vi "UI_Export Setting.vi"(8 "error in (no error)":errorcluster) -> (0 "error out":errorcluster)   [LabVIEW 2015, in "ConfigHelper.lvlib"]
uses:
  ConfigHelper.lvlib
  Control_Export File Setup.ctl
  Control_UI_Export Setting.ctl
  Control_UI_Export Setting State.ctl
  <vilib>/addons/PointValueMap/controls/PointMap.ctl
  <vilib>/addons/PointValueMap/PointValueMap.lvlib
panel:
  in  "Export File Setup":T1
  in  "Copy Device":bool
  in  "Save Button":bool
  in  "Import from TDMS":bool
  in  "Remove Channel":bool
  in  "Add Channel":bool
  in  "Remove Device":bool
  in  "Add Device":bool
  in  "Channel Names":i32[](listbox)
  in  "Device Name":i32[](listbox)
  in  "OK Button":bool
  in  "Cancel Button":bool
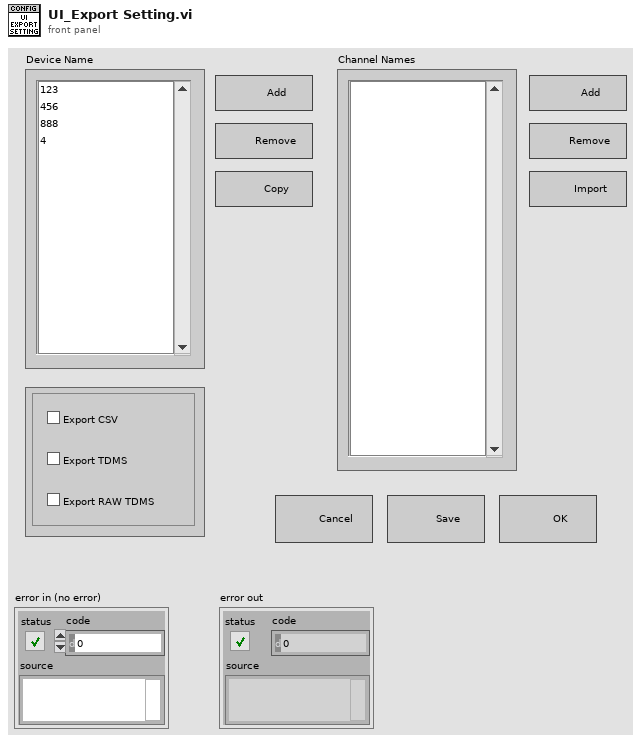
[diagram p1: front panel]
types:
  T1 = typedef "ConfigHelper.lvlib/Control_Export File Setup.ctl" = cluster{"CSV":bool, "TDMS":bool, "RAW TDMS":bool}
  T2 = typedef "ConfigHelper.lvlib/Control_UI_Export Setting State.ctl" = enum16{"Init", "Wait", "Exit", "Write to File", "Read from PVM", "Write to PVM", "Update Device", "Add Device", "Remove Device", "Copy Device", "Update Channel", "Add Channel", "Remove Channel", "Import from TDMS"}
  T3 = typedef "ConfigHelper.lvlib/Control_UI_Export Setting.ctl" = cluster{"State":T2, "Map":T4, "Device Name":refnum<vi>, "Channel Name":refnum<vi>, "File Setup":refnum<vi>, "Name":string, "Devices Selected":i32[]}
  T4 = typedef "PointValueMap.lvlib/PointMap.ctl" = refnum<data-value>
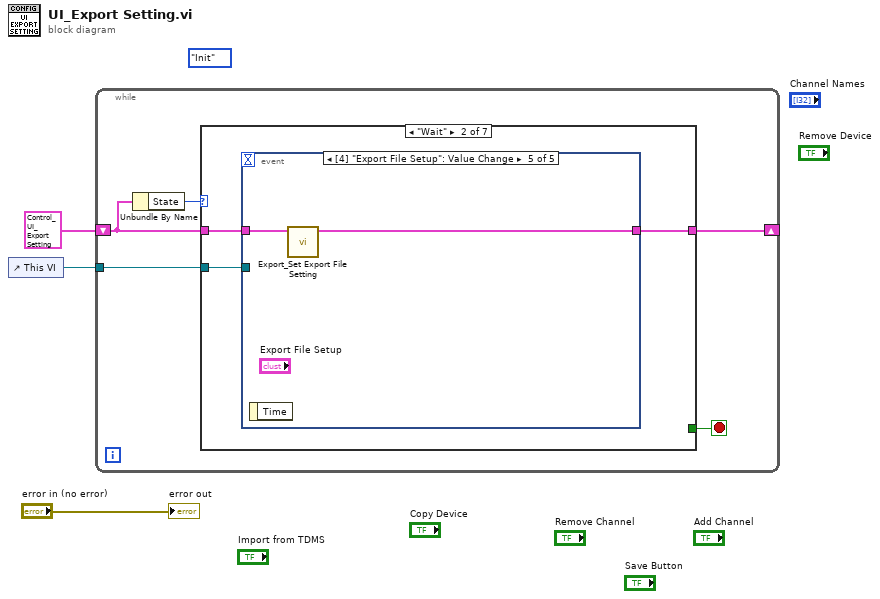
[diagram p0: block diagram]
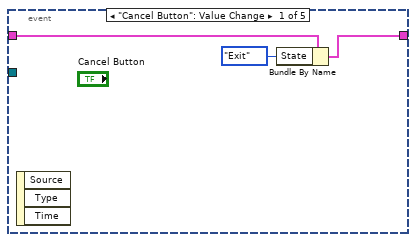
[diagram p3: hidden frame]
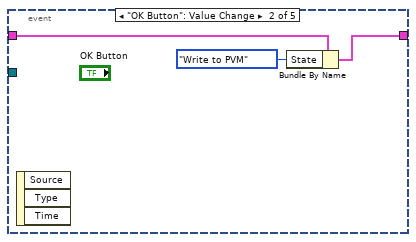
[diagram p4: hidden frame]
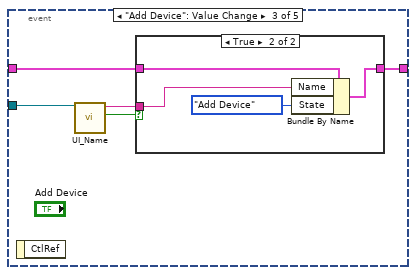
[diagram p5: hidden frame]
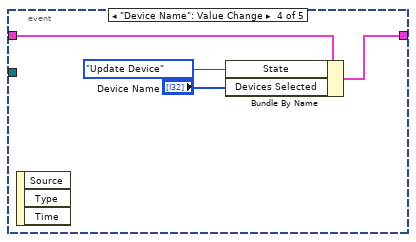
[diagram p7: hidden frame]
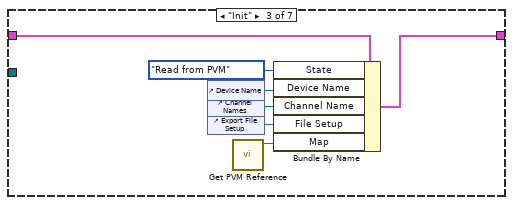
[diagram p8: hidden frame]
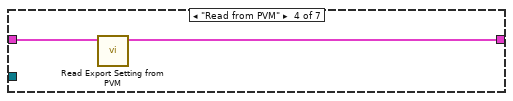
[diagram p9: hidden frame]
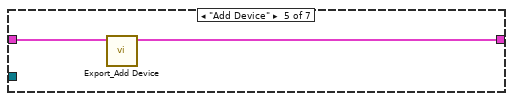
[diagram p10: hidden frame]
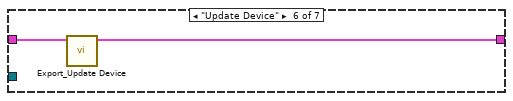
[diagram p11: hidden frame]
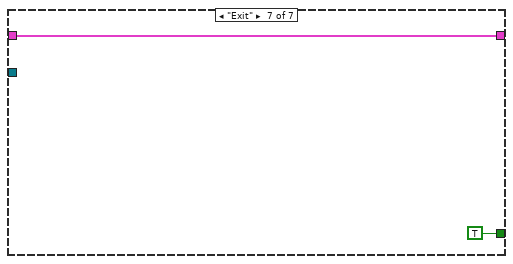
[diagram p12: hidden frame]
diagram:
  (unwired) Control_UI_Export_Setting_State."Init" ("State")
  n1 = control-ref of="This VI"() -> (w1:refnum<vi>)
  n2 = while {
    shift-right: [w7] -> _
    shift-left: T3 {"State"=enum."Init", "Map"=refnum, "Device Name"=refnum, "Channel Name"=refnum, "File Setup"=refnum, "Name"="", "Devices Selected"=[]} ("UI Export Setting") -> [w8]
    tunnel: w1 -> [w4]
    stop <- w6 stop-if-true
    n3 = Unbundle By Name(w8) -> ("State"=w5:T2)
    n4 = case shown="\"Wait\"" w5 {
      tunnel: w8 -> [w9 w12 w41 w43 w45 w47 w49]
      tunnel: [w9 w11 w40 w42 w44 w46 w49] -> w7
      tunnel: [_ _ _ _ _ _ TRUE] -> w6
      tunnel: w4 -> [_ w10 _ _ _ _ _]
      frame Default {
      }
      frame "Wait" {
        n5 = event shown="[4] \"Export File Setup\": Value Change" {
          selector: _ -> [_ _ _ _ _]
          dyn-events: _ -> [_ _ _ _ _]
          timeout: _ -> [_ _ _ _ _]
          tunnel: w12 -> [w15 w18 w21 w32 w34]
          tunnel: [w14 w17 w20 w30 w33] -> w11
          tunnel: w10 -> [_ _ w19 _ _]
          event "Cancel Button": Value Change {
            n6 = event-data() -> ()  [unwired: 1 in, 3 out]
            n7 = Bundle By Name(cluster=w15, "State"=Control_UI_Export_Setting_State."Exit") -> (w14:T3)
          }
          event "OK Button": Value Change {
            n8 = event-data() -> ()  [unwired: 1 in, 3 out]
            n9 = Bundle By Name(cluster=w18, "State"=Control_UI_Export_Setting_State."Write to PVM") -> (w17:T3)
          }
          event "Add Device": Value Change {
            n10 = event-data() -> ()  [unwired: 1 in, 1 out]
            n11 = call "UI_Name.vi"("Main VI"=w19) -> ("Vaild?"=w23:bool, "Name Output"=w22:string)  [unwired: 9 in]
            n12 = case shown="True" w23 {
              tunnel: w22 -> [_ w27]
              tunnel: w21 -> [w24 w28]
              tunnel: [w24 w26] -> w20
              frame False {
              }
              frame True {
                n13 = Bundle By Name(cluster=w28, "Name"=w27, "State"=Control_UI_Export_Setting_State."Add Device") -> (w26:T3)
              }
            }
          }
          event "Device Name": Value Change {
            n14 = event-data() -> ()  [unwired: 1 in, 3 out]
            n15 = Bundle By Name(cluster=w32, "State"=Control_UI_Export_Setting_State."Update Device", "Devices Selected"="Device Name") -> (w30:T3)
          }
          event Value Change {
            n16 = event-data() -> ()  [unwired: 1 in, 1 out]
            n17 = call "Export_Set Export File Setting.vi"("Export Setting in"=w34) -> ("Export Setting out"=w33:T3)  [unwired: 10 in]
          }
        }
      }
      frame "Init" {
        n18 = control-ref of="Device Name"() -> (w38:refnum<vi>)
        n19 = control-ref of="Channel Names"() -> (w37:refnum<vi>)
        n20 = control-ref of="Export File Setup"() -> (w36:refnum<vi>)
        n21 = call "Get PVM Reference.vi"() -> ("Map Out"=w35:T4)  [unwired: 10 in, 1 out]
        n22 = Bundle By Name(cluster=w41, "State"=Control_UI_Export_Setting_State."Read from PVM", "Device Name"=w38, "Channel Name"=w37, "File Setup"=w36, "Map"=w35) -> (w40:T3)
      }
      frame "Read from PVM" {
        n23 = call "Read Export Setting from PVM.vi"("Export Setting in"=w43) -> ("Export Setting out"=w42:T3)  [unwired: 10 in]
      }
      frame "Add Device" {
        n24 = call "Export_Add Device.vi"("Export Setting in"=w45) -> ("Export Setting out"=w44:T3)  [unwired: 10 in]
      }
      frame "Update Device" {
        n25 = call "Export_Update Device.vi"("Export Setting in"=w47) -> ("Export Setting out"=w46:T3)  [unwired: 10 in]
      }
      frame "Exit" {
      }
    }
  }
  "error out" <- "error in (no error)"
